vi "TestFindFaces_LV18Nodes.vi"() -> ()   [LabVIEW 2018]
uses:
  <vilib>/ptbypt/NI_PtbyPt.lvlib
panel:
  out "Mean Execution Time (s)":dbl
  in  "stop":bool
  out "Execution Time":dbl(graph)
  out "image with faces":picture
  # "This VI Demonstrates using the LabVIEW 2018 Python Nodes with OpenCV to do simple facial recognition on an image and benchmarks its execution time for comparison with other methods of communicating with Python in LabVIEW. \nIt will read an image file and draw a box around the face."
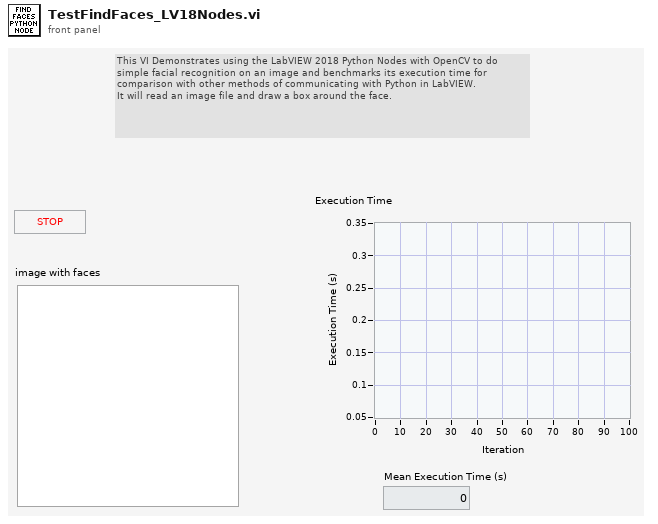
[diagram p1: front panel]
types:
  T1 = typedef "imagedata.ctl" = cluster{"image type":i32, "image depth":i32, "image":u8[], "mask":u8[], "colors":u32[], "Rectangle":cluster{"left":i16, "top":i16, "right":i16, "bottom":i16}}
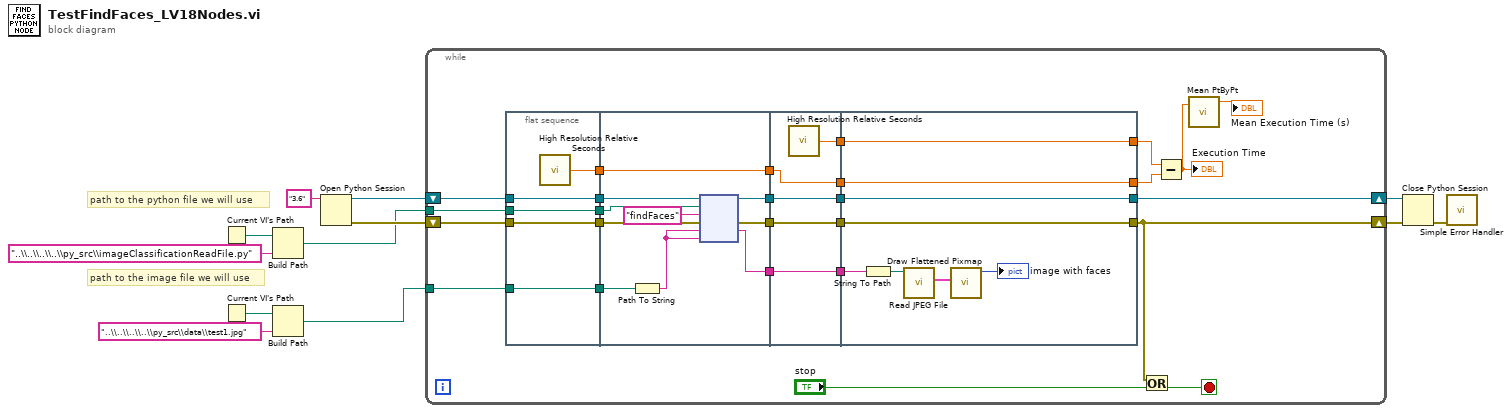
[diagram p0: block diagram]
diagram:
  # "path to the image file we will use"
  # "path to the python file we will use"
  n1 = Current VI's Path() -> (path=w6:path)
  n2 = Current VI's Path() -> (path=w3:path)
  n3 = Build Path(base path=w6, name or relative path="..\\..\\..\\..\\py_src\\imageClassificationReadFile.py") -> (appended path=w4:path)
  n4 = Build Path(base path=w3, name or relative path="..\\..\\..\\..\\py_src\\data\\test1.jpg") -> (appended path=w1:path)
  n5 = Open Python Session(python version="3.6" ("Python version")) -> (session out=w12:refnum<k35>, error out=w11:errorcluster)  [unwired: 2 in]
  n6 = while {
    shift-right: [w36] -> w9
    shift-left: w12 -> [w38]
    shift-right: [w29] -> w8
    shift-left: w11 -> [w37]
    tunnel: w4 -> [w24]
    tunnel: w1 -> [w23]
    stop <- w30 stop-if-true
    n7 = flat-sequence {
      tunnel: w23 -> [w40]
      tunnel: w24 -> [w41]
      tunnel: w37 -> [w42]
      tunnel: w38 -> [w43]
      tunnel: [w43] -> w20
      tunnel: [w42] -> w19
      tunnel: [w41] -> w18
      tunnel: [w40] -> w17
      tunnel: [w39] -> w15
      tunnel: [w48] -> w34
      tunnel: [w52] -> w33
      tunnel: [w46] -> w21
      tunnel: w20 -> [w53]
      tunnel: w19 -> [w49]
      tunnel: w18 -> [w51]
      tunnel: w17 -> [w47]
      tunnel: [w45] -> w16
      tunnel: w15 -> [w45]
      tunnel: w34 -> [w58]
      tunnel: w33 -> [w57]
      tunnel: [w58] -> w28
      tunnel: [w57] -> w27
      tunnel: [w56] -> w26
      tunnel: [w54] -> w25
      tunnel: [w55] -> w22
      tunnel: w21 -> [w55]
      tunnel: w16 -> [w54]
      tunnel: [w63] -> w31
      tunnel: [w64] -> w32
      tunnel: [w65] -> w36
      tunnel: [w66] -> w29
      tunnel: w28 -> [w66]
      tunnel: w27 -> [w65]
      tunnel: w26 -> [w64]
      tunnel: w25 -> [w63]
      tunnel: w22 -> [w61]
      frame #0 {
        n8 = call <vilib>:"High Resolution Relative Seconds.vi"() -> ("relative seconds"=w39:dbl)
      }
      frame #1 {
        n9 = Path To String(path=w47) -> (string=w44:string)
        n10 = node(w53, w51, "findFaces" ("function name"), w49, w44, w44) -> (w52:refnum<k35>, w48:errorcluster, w46:string)  [unwired: 1 in, 2 out]
      }
      frame #2 {
        n11 = call <vilib>:"High Resolution Relative Seconds.vi"() -> ("relative seconds"=w56:dbl)
      }
      frame #3 {
        n12 = String To Path(string=w61) -> (path=w60:path)
        n13 = call <vilib>:"Read JPEG File.vi"("path to JPEG file"=w60) -> ("image data"=w59:T1)  [unwired: 8 in, 2 out]
        n14 = call <vilib>:"Draw Flattened Pixmap.vi"("image data"=w59) -> ("new picture"=→"image with faces":picture)  [unwired: 8 in]
      }
    }
    n15 = Or(x=w29, y="stop") -> (x .or. y?=w30:bool)
    n16 = Subtract(x=w32, y=w31) -> (x-y=w13:dbl)
    "Execution Time" <- w13
    n17 = call <vilib>:"Mean PtByPt.vi"("x"=w13) -> ("mean"=→"Mean Execution Time (s)":dbl)  [unwired: 3 in, 1 out]
  }
  n18 = Close Python Session(session in=w9, error in=w8) -> (11:w10:errorcluster)
  n19 = call <vilib>:"Simple Error Handler.vi"("error in (no error)"=w10) -> ()  [unwired: 4 in, 5 out]
